vi "Teleop.vi"(10 "Match Info":T2={"Autonomous Elapsed Seconds"=0.0, "TeleOp Elapsed Seconds"=0.0, "Disabled Elapsed Seconds"=0.0, "Visited Autonomous"=FALSE, "Visited TeleOp"=FALSE, "Visited Disabled"=FALSE, "Autonomous Settings"={"Autonomous Style"=enum."Independent", "VI Refnum"=refnum}}, 11 "Call Context":T3) -> ()   [LabVIEW 2016]
doc: "This VI is called for each TeleOp packet received from the DS where the robot is not disabled. It is often used to read from the joysticks and update I/O or to update setpoints for timed control loops. It should complete and return within 20 milliseconds or it may miss DS packets."
uses:
  <vilib>/Rock Robotics/WPI/DriverStation/WPI_DriverStationDerivedRobotMode.ctl
  <vilib>/Rock Robotics/WPI/DriverStation/WPI_DriverStationMatch Info.ctl
  <vilib>/Rock Robotics/WPI/Utilities/WPI_GetSetVariantRefNum.vi
  Robot Global Data.vi
  <vilib>/Rock Robotics/WPI/Solenoid/Deprecated/WPI_SolenoidSetBool.vi
  <vilib>/addons/control/pid/pid.llb/PID (DBL).vi
  navX Library v2/navX Library v2.lvlib
  <vilib>/addons/control/pid/NI_PID_pid.lvlib
panel:
  in  "Mode":bool
  in  "output range":cluster{"output high":dbl, "output low":dbl}={"output high"=100.0, "output low"=-100.0} {"output low" format="%.2f"; "output high" format="%.2f"}
  in  "PID gains":T1={"proportional gain (Kc)"=1.0, "integral time (Ti, min)"=0.01, "derivative time (Td, min)"=0.0} {"derivative time (Td, min)" format="%.3f"; "integral time (Ti, min)" format="%.3f"; "proportional gain (Kc)" format="%.3f"}
  out "Left":dbl(graph)
  out "Right":dbl(graph)
  out "Encoder Right":dbl(graph)
  out "Encoder Left":dbl(graph)
  in  "Speed":dbl=0.5 format="%#_13g"
  out "Out Left":dbl(graph)
  out "Out Right":dbl(graph)
  out "Shooter":cluster{"Sensor Velocity":dbl, dbl, dbl}(graph)
  in  "ShooterRPM":dbl
  in  "P":dbl=0.5 format="%#_13g"
  in  "I":dbl format="%#_13g"
  in  "D":dbl format="%#_13g"
  in  "F":dbl=0.005212 format="%#_13g"
  in  "I Zone":dbl format="%#_13g"
  in  "Ramp Rate":dbl format="%#_13g"
  # "False = PID On\nTrue = PID Off\nDon't switch!!!"
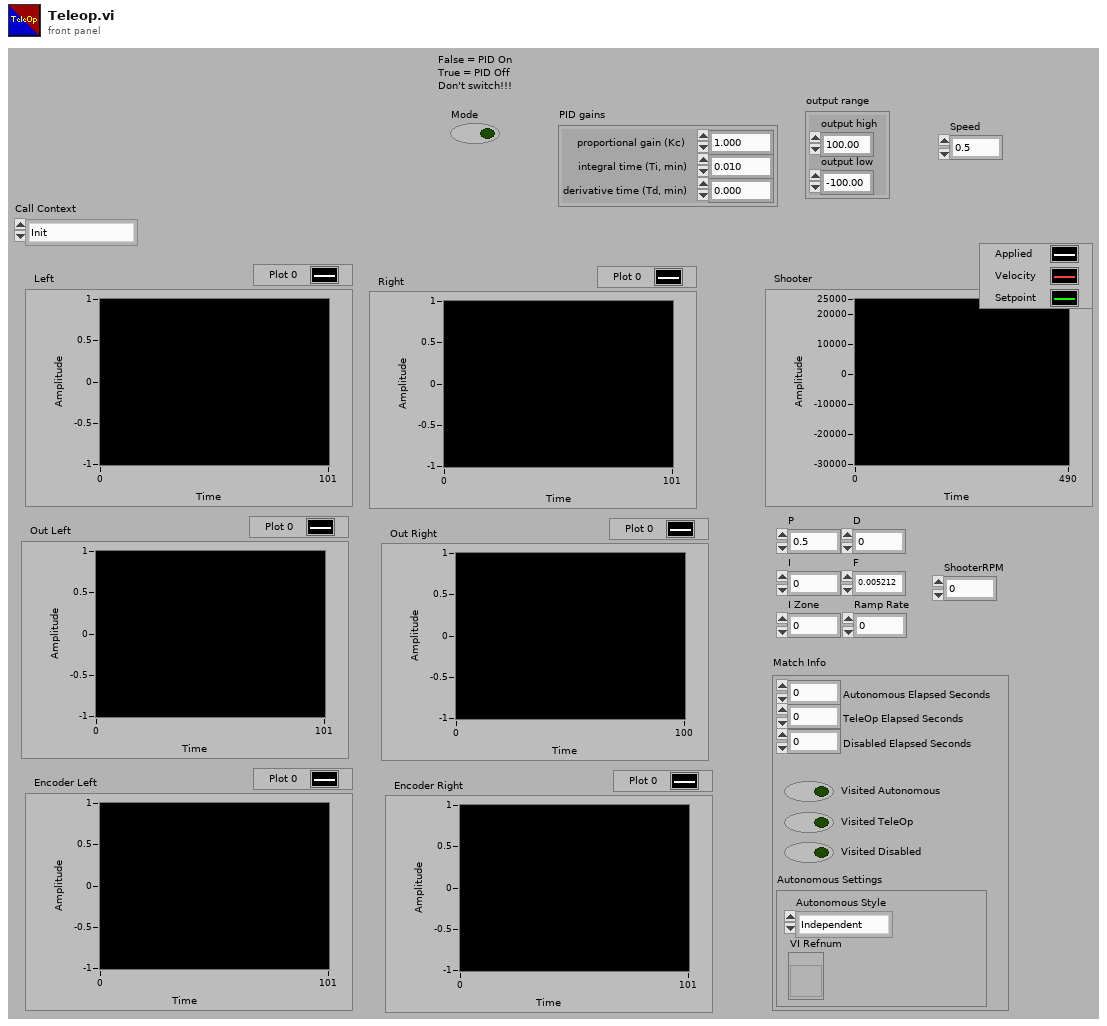
[diagram p1: front panel]
types:
  T1 = cluster{"proportional gain (Kc)":dbl, "integral time (Ti, min)":dbl, "derivative time (Td, min)":dbl}
  T2 = typedef "WPI_DriverStationMatch Info.ctl" = cluster{"Autonomous Elapsed Seconds":dbl, "TeleOp Elapsed Seconds":dbl, "Disabled Elapsed Seconds":dbl, "Visited Autonomous":bool, "Visited TeleOp":bool, "Visited Disabled":bool, "Autonomous Settings":cluster{"Autonomous Style":enum16{"Iterative", "Independent"}, "VI Refnum":refnum<vi>}}
  T3 = typedef "WPI_DriverStationDerivedRobotMode.ctl" = enum16{"Init", "Execute", "Stop"}
  T4 = typedef "WPI_SolenoidDevRef.ctl" = cluster{"DevStatus":errorcluster, "Pneumatics Control Module":u8, "Forward Solenoid Channel":T5, "Reverse Solenoid Channel":T5}
  T5 = typedef "WPI_SolenoidChannel.ctl" = enum8{"Solenoid 0", "Solenoid 1", "Solenoid 2", "Solenoid 3", "Solenoid 4", "Solenoid 5", "Solenoid 6", "Solenoid 7", "Invalid"}
  T6 = typedef "WPI_JoystickDevRef.ctl" = cluster{"Device":T7}
  T7 = typedef "WPI_JoystickDeviceEnum.ctl" = enum16{"USB 0", "USB 1", "USB 2", "USB 3", "USB 4", "USB 5"}
  T8 = cluster{"Buttons[0]":bool, "Buttons[1]":bool, "Buttons[2]":bool, "Buttons[3]":bool, "Buttons[4]":bool, "Buttons[5]":bool, "Buttons[6]":bool, "Buttons[7]":bool, "Buttons[8]":bool}
  T9 = cluster{"Axes[0]":dbl, "Axes[1]":dbl, "Axes[2]":dbl, "Axes[3]":dbl, "Axes[4]":dbl, "Axes[5]":dbl, "Axes[6]":dbl, "Axes[7]":dbl, "Axes[8]":dbl}
  T10 = typedef "navX Library v2.lvlib/Z900_navX_DeviceTypeDef.ctl" = cluster{"Interface":cluster{"Protocol":T11, "Update Rate (4Hz-100Hz)":u8, "navX Open TypeDef":variant}, "Notify Packet":refnum<notifier>, "Loop VI Refnum":refnum<vi>, "Ready to Close Occurrence Refnum":refnum<k4>}
  T11 = typedef "navX Library v2.lvlib/Z900_navX_ProtocolTypeDef.ctl" = enum16{"SERIAL", "I2C", "SPI"}
  T12 = cluster{"Velocity X":dbl, "Velocity Y":dbl, "Velocity Z":dbl, "Displacement X":dbl, "Displacement Y":dbl, "Displacement Z":dbl}
  T13 = cluster{"LinearAcceleration X":dbl, "LinearAcceleration Y":dbl, "LinearAcceleration Z":dbl}
  T14 = cluster{"Quat W":dbl, "Quat X":dbl, "Quat Y":dbl, "Quat Z":dbl}
  T15 = cluster{"Yaw":dbl, "Roll":dbl, "Pitch":dbl, "Heading":dbl, "Fused Heading":dbl}
  T16 = cluster{"Velocity X":dbl, "Velocity Y":dbl, "Velocity Z":dbl, "Displacement X":dbl, "Displacement Y":dbl, "Displacement Z":dbl, "LinearAcceleration X":dbl, "LinearAcceleration Y":dbl, "LinearAcceleration Z":dbl, "Quat W":dbl, "Quat X":dbl, "Quat Y":dbl, "Quat Z":dbl, "Yaw":dbl, "Roll":dbl, "Pitch":dbl}
  T17 = typedef "WPI_MotorControlDeviceRef.ctl" = cluster{"DeviceStatus":errorcluster, "Type":T18, "PWM":cluster{"PWM Channel":T19, "DeadBand":T20}, "CAN":cluster{"Device Number":u8, "SetOutput VI Ref":variant, "GetOutput VI Ref":variant, "Enable VI Ref":variant, "Disable VI Ref":variant, "Data":variant}, "Invert":bool}
  T18 = typedef "WPI_MotorControlType.ctl" = enum16{"PWM", "CAN"}
  T19 = typedef "FPGA_DIOPWMChannel.ctl" = enum8{"PWM 0", "PWM 1", "PWM 2", "PWM 3", "PWM 4", "PWM 5", "PWM 6", "PWM 7", "PWM 8", "PWM 9", "PWM MXP 0", "PWM MXP 1", "PWM MXP 2", "PWM MXP 3", "PWM MXP 4", "PWM MXP 5", "PWM MXP 6", "PWM MXP 7", "PWM MXP 8", "PWM MXP 9", "Invalid"}
  T20 = typedef "WPI_PWMDeadband.ctl" = cluster{"Name":string, "maxPositivePwm":i32, "minPositivePwm":i32, "centerPwm":i32, "maxNegativePwm":i32, "minNegativePwm":i32, "angularRange":u16}
  T21 = typedef "WPI_CANTalonSRX_GlobalStatus.ctl" = cluster{"Applied Throttle":dbl, "Module Enabled":bool, "CAN Error":errorcluster, "Closed Loop Error":dbl, "Forward Limit Switch Closed":bool, "Reverse Limit Switch Closed":bool, "Sensor Position":dbl, "Sensor Velocity":dbl, "Current":dbl, "Sticky Fault - Over Temp":bool, "Sticky Fault - Under Voltage":bool, "Sticky Fault - Forward Limit":bool, "Sticky Fault - Reverse Limit":bool, "Sticky Fault - Forward Soft Limit":bool, "Sticky Fault - Reverse Soft Limit":bool, "Brake is Enabled":bool, "Encoder Position":dbl, "Encoder Velocity":dbl, "Encoder Index Count":dbl, "Encoder A Pin State":bool, "Encoder B Pin State":bool, "Encoder Index Pin State":bool, "Analog In":dbl, "Analog In Velocity":dbl, "Temperature (C)":dbl, "Battery Voltage":dbl, "Control 5 Is Supported":bool, "Current Profile Slot Select":dbl, "Pos Div 8":bool, "Vel Div 4":bool, "Pulse Width Position":i32, "Pulse Width Velocity":i32, "Pulse Width Rise To Rise (us)":i32, "Pulse Width Rise To Fall (us)":i32, "Mot Prof Active Is Under Run":bool, "Mot Prof Active Has Under Run":bool, "Mot Prof Active Is Last":bool, "Mot Prof Active Velocity Only":bool, "Mot Prof Active Is Valid":bool, "Mot Prof Buffer Is Full":bool, "Mot Prof Active Profile Slot Select":i32, "Mot Prof NextID":i32, "Mot Prof Count":i32, "Mot Prof Active Velocity":dbl, "Mot Prof Active Position":dbl, "Mot Prof Output Enable":i32}
  T22 = cluster{dbl, "Sensor Velocity":dbl, "ShooterRPM":dbl}
  T23 = typedef "WPI_RobotDriveDevRef.ctl" = cluster{"DevStatus":errorcluster, "Motors[]":T17[], "Square Inputs":bool, "Max Output":dbl}
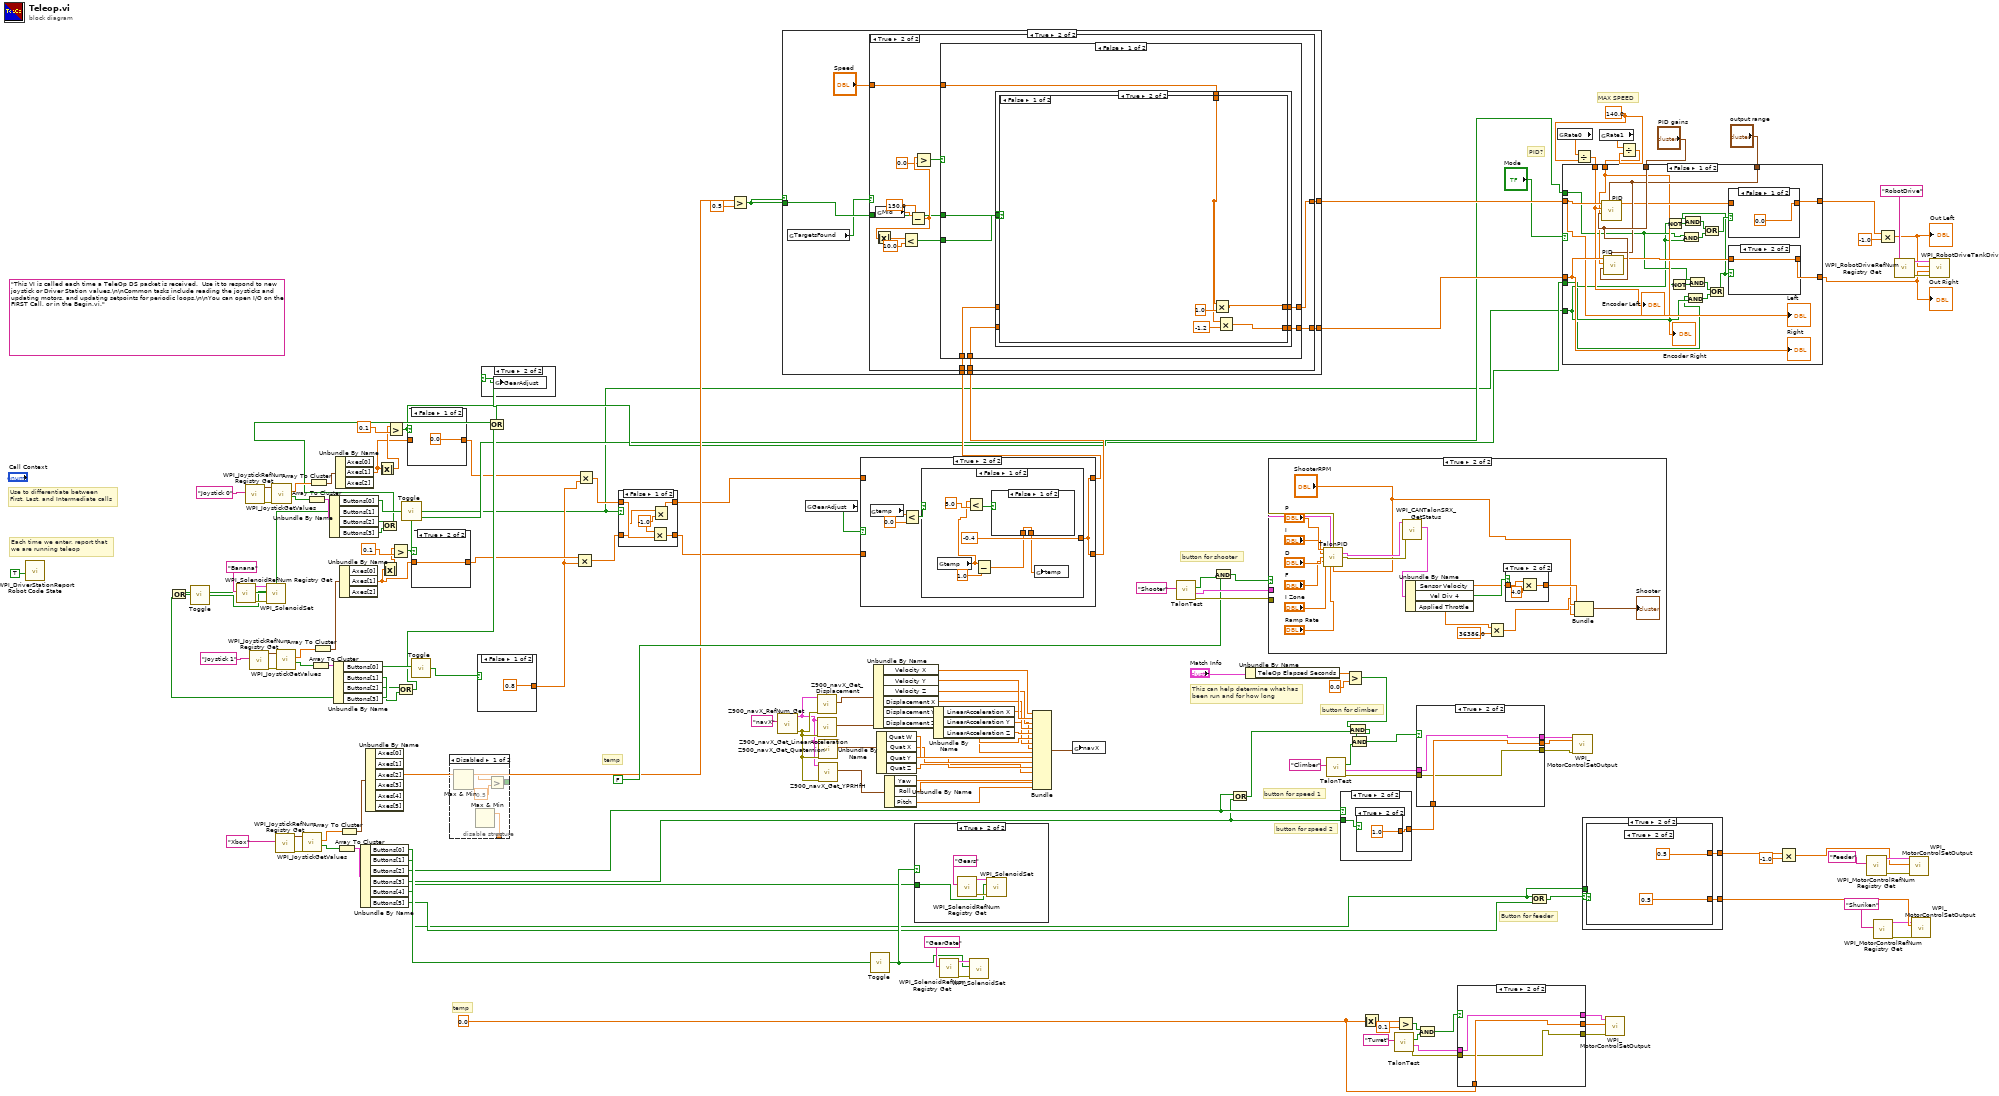
[diagram p0: block diagram]
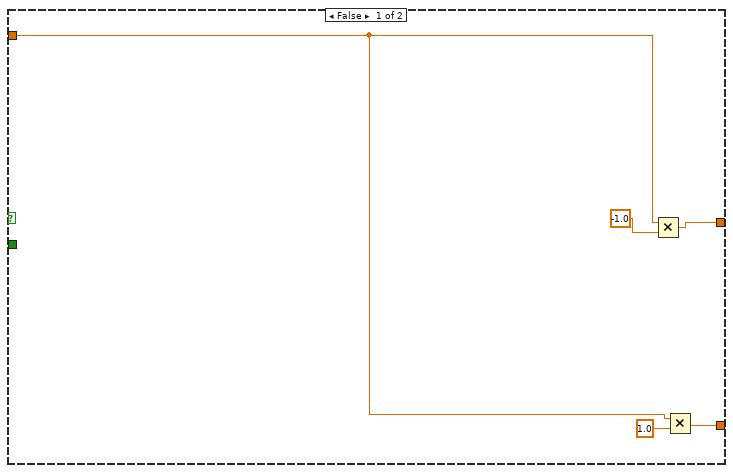
[diagram p3: hidden frame]
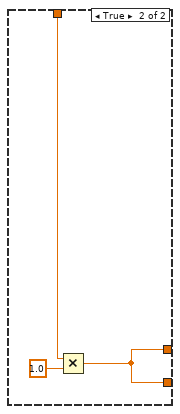
[diagram p5: hidden frame]
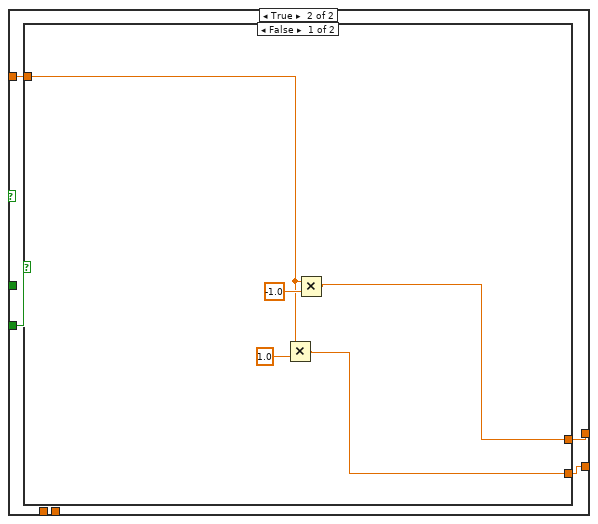
[diagram p6: hidden frame]
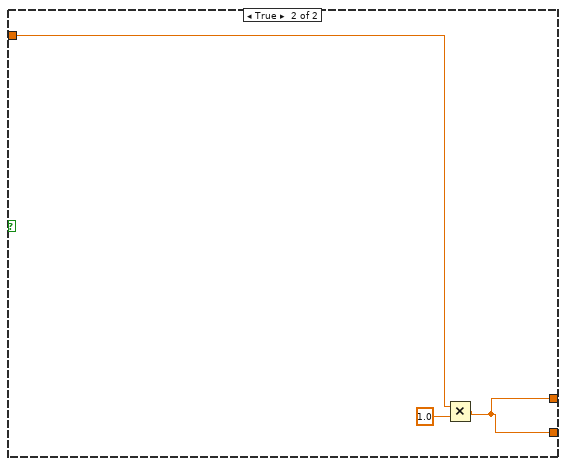
[diagram p7: hidden frame]
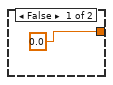
[diagram p8: hidden frame]
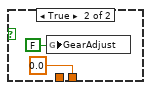
[diagram p14: hidden frame]
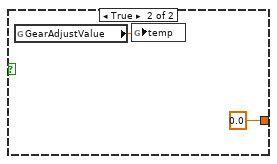
[diagram p15: hidden frame]
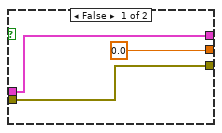
[diagram p16: hidden frame]
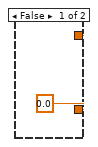
[diagram p18: hidden frame]
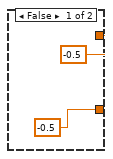
[diagram p19: hidden frame]
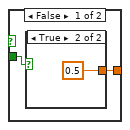
[diagram p20: hidden frame]
diagram:
  w21 = 140.0
  w34 = 0.0
  (unwired) "This VI is called each time a TeleOp DS packet is received.  Use it to respond to new joystick or Driver Station values.\n\nCommon tasks include reading the joysticks and updating motors, and updating setpoints for periodic loops.\n\nYou can open I/O on the FIRST Call, or in the Begin.vi."
  # "MAX SPEED"
  # "PID?"
  # "temp"
  # "temp"
  # "Button for feeder"
  # "button for speed 2"
  # "button for speed 1"
  # "button for climber"
  # "button for shooter"
  # "Each time we enter, report that\nwe are running teleop"
  # "Use to differentiate between\nFirst, Last, and Intermediate calls"
  # "This can help determine what has\nbeen run and for how long"
  n1 = call <vilib>:"WPI_DriverStationReport Robot Code State.vi"("TeleOp"=TRUE ("Autonomous")) -> ()  [unwired: 10 in, 1 out]
  n2 = call <vilib>:"WPI_SolenoidRefNum Registry Get.vi"("refnum name"="Banana") -> ("error out"=w59:errorcluster, "SolenoidDevRef"=w58:T4)  [unwired: 9 in]
  n3 = call <vilib>:"WPI_JoystickRefNum Registry Get.vi"("refnum name"="Joystick 0") -> ("error out"=w155:errorcluster, "JoystickDevRef"=w154:T6)  [unwired: 9 in]
  n4 = call <vilib>:"WPI_JoystickRefNum Registry Get.vi"("refnum name"="Joystick 1") -> ("error out"=w147:errorcluster, "JoystickDevRef"=w146:T6)  [unwired: 9 in]
  n5 = call <vilib>:"WPI_JoystickGetValues.vi"("error in (no error)"=w155, "JoystickDevRef"=w154) -> ("Buttons"=w151:bool[], "Axes"=w152:dbl[])  [unwired: 5 in, 3 out]
  n6 = call <vilib>:"WPI_JoystickRefNum Registry Get.vi"("refnum name"="Xbox") -> ("error out"=w88:errorcluster, "JoystickDevRef"=w87:T6)  [unwired: 9 in]
  n7 = call <vilib>:"WPI_JoystickGetValues.vi"("error in (no error)"=w147, "JoystickDevRef"=w146) -> ("Buttons"=w143:bool[], "Axes"=w144:dbl[])  [unwired: 5 in, 3 out]
  n8 = call <vilib>:"WPI_JoystickGetValues.vi"("error in (no error)"=w88, "JoystickDevRef"=w87) -> ("Buttons"=w84:bool[], "Axes"=w85:dbl[])  [unwired: 5 in, 3 out]
  n9 = Array To Cluster(array=w151) -> (cluster=w149:T8)
  n10 = Array To Cluster(array=w152) -> (cluster=w150:T9)
  n11 = Array To Cluster(array=w143) -> (cluster=w141:T8)
  n12 = Array To Cluster(array=w144) -> (cluster=w142:T9)
  n13 = Unbundle By Name(w149) -> ("Buttons[0]"=w135:bool, "Buttons[1]"=w55:bool, "Buttons[2]"=w40:bool, "Buttons[3]"=w39:bool)
  n14 = Unbundle By Name(w141) -> ("Buttons[0]"=w134:bool, "Buttons[1]"=w54:bool, "Buttons[2]"=w42:bool, "Buttons[3]"=w41:bool)
  n15 = Or(x=w55, y=w54) -> (x .or. y?=w56:bool)
  n16 = call "Toggle.vi"("Input"=w56) -> ("Output"=w53:bool)
  n17 = call-poly <vilib>:"WPI_SolenoidSet.vi"("error in (no error)"=w59, "Value"=w53, "SolenoidDevRef"=w58) -> ()  [unwired: 7 in, 2 out]
  n18 = Unbundle By Name(w150) -> ("Axes[1]"=w136:dbl)  [unwired: 2 out]
  n19 = Array To Cluster(array=w84) -> (cluster=w82:T8)
  n20 = Unbundle By Name(w142) -> ("Axes[1]"=w138:dbl)  [unwired: 2 out]
  n21 = Array To Cluster(array=w85) -> (cluster=w83:T9)
  n22 = Unbundle By Name(w82) -> ("Buttons[0]"=w81:bool, "Buttons[1]"=w80:bool, "Buttons[2]"=w79:bool, "Buttons[3]"=w78:bool, "Buttons[4]"=w75:bool, "Buttons[5]"=w76:bool)
  n23 = Unbundle By Name(w83) -> ("Axes[2]"=w32:dbl)  [unwired: 5 out]
  n24 = Absolute Value(x=w136) -> (abs(x)=w137:dbl)
  n25 = Or(x=w40, y=w39) -> (x .or. y?=w38:bool)
  n26 = Absolute Value(x=w138) -> (abs(x)=w139:dbl)
  n27 = Greater?(x=w137, y=0.1 ("x")) -> (0:w11:bool)
  n28 = Greater?(x=w139, y=0.1 ("x")) -> (0:w10:bool)
  n29 = Or(x=w42, y=w41) -> (x .or. y?=w37:bool)
  n30 = call "Toggle.vi"("Input"=w135) -> ("Output"=w1:bool)
  n31 = case shown="False" w11 {
    tunnel: w136 -> [_ w158]
    tunnel: [0.0 w158] -> w6
    frame False {
    }
    frame True {
    }
  }
  n32 = case shown="True" w10 {
    tunnel: w138 -> [_ w160]
    tunnel: [0.0 w160] -> w8
    frame False {
    }
    frame True {
    }
  }
  n33 = call "Toggle.vi"("Input"=w134) -> ("Output"=w133:bool)
  n34 = disable-structure shown="Disabled" {
    disable-tunnel: [w162 _] -> _
    disable-tunnel: [w161 _] -> _
    frame Disabled {
      n35 = Max & Min() -> (max(x,y)=w164:dbl)  [unwired: 2 in, 1 out]
      n36 = Max & Min() -> (max(x,y)=w161:dbl)  [unwired: 2 in, 1 out]
      n37 = Greater?(x=w164, y=0.5) -> (0:w162:bool)
    }
    frame Enabled {
    }
  }
  n38 = case shown="False" w133 {
    tunnel: [0.8 1.0] -> w7
    frame False {
    }
    frame True {
    }
  }
  n39 = Or(x=w38, y=w37) -> (x .or. y?=w35:bool)
  n40 = case shown="True" w35 {
    selector: w35 -> [_ w167]
    frame False {
    }
    frame True {
      n41 = global write "Robot Global Data.vi" "GearAdjust"(w167) -> ()
    }
  }
  n42 = Multiply(x=w8, y=w7) -> (x*y=w4:dbl)
  n43 = Multiply(x=w6, y=w7) -> (x*y=w5:dbl)
  n44 = case shown="False" w1 {
    tunnel: w5 -> [w169 w174]
    tunnel: w4 -> [w168 w173]
    tunnel: [w172 w174] -> w3
    tunnel: [w171 w173] -> w2
    frame False {
      w170 = -1.0
      n45 = Multiply(x=w170, y=w169) -> (x*y=w171:dbl)
      n46 = Multiply(x=w168, y=w170) -> (x*y=w172:dbl)
    }
    frame True {
    }
  }
  n47 = Greater?(x=w32, y=0.5) -> (0:w9:bool)
  n48 = call "Z900_navX_RefNum_Get.vi"("refnum name"="navX") -> ("error out"=w131:errorcluster, "navX Device"=w130:T10)  [unwired: 9 in]
  n49 = global read "Robot Global Data.vi" "GearAdjust"() -> (w36:bool)
  n50 = call "Z900_navX_Get_Displacement.vi"("error in (no error)"=w131, "navX Device"=w130) -> ("Displacement"=w126:T12)  [unwired: 6 in, 3 out]
  n51 = call "Z900_navX_Get_LinearAcceleration.vi"("error in (no error)"=w131, "navX Device"=w130) -> ("Linear Acceleration"=w127:T13)  [unwired: 6 in, 3 out]
  n52 = call "Z900_navX_Get_Quaternion.vi"("error in (no error)"=w131, "navX Device"=w130) -> ("Quaternion"=w128:T14)  [unwired: 6 in, 3 out]
  n53 = call "Z900_navX_Get_YPRHfH.vi"("error in (no error)"=w131, "navX Device"=w130) -> ("YRPHfH"=w129:T15)  [unwired: 6 in, 3 out]
  n54 = case shown="True" w36 {
    tunnel: w3 -> [w176 _]
    tunnel: w2 -> [w175 _]
    tunnel: [w176 w177] -> w27
    tunnel: [w175 w177] -> w26
    frame False {
    }
    frame True {
      n55 = global read "Robot Global Data.vi" "temp"() -> (w180:dbl)
      n56 = Less?(x=w180, y=0.0) -> (x < y?=w178:bool)
      n57 = case shown="False" w178 {
        tunnel: [-0.4 0.0] -> w177
        frame False {
          n58 = global read "Robot Global Data.vi" "temp"() -> (w183:dbl)
          n59 = Less?(x=w183, y=5.0 ("x")) -> (x < y?=w184:bool)
          n60 = Subtract(x=w183, y=1.0) -> (x-y=w181:dbl)
          n61 = case shown="False" w184 {
            tunnel: [w188 0.0] -> w182
            tunnel: w181 -> [w188 _]
            frame False {
            }
            frame True {
              n62 = global write "Robot Global Data.vi" "GearAdjust"(FALSE) -> ()
            }
          }
          n63 = global write "Robot Global Data.vi" "temp"(w182) -> ()
        }
        frame True {
          n64 = global read "Robot Global Data.vi" "GearAdjustValue"() -> (w192:dbl)
          n65 = global write "Robot Global Data.vi" "temp"(w192) -> ()
        }
      }
    }
  }
  n66 = case shown="True" w9 {
    tunnel: w27 -> [w194 w201]
    tunnel: w26 -> [w193 w200]
    tunnel: w9 -> [_ w198]
    tunnel: [w194 w197] -> w17
    tunnel: [w193 w196] -> w16
    frame False {
    }
    frame True {
      n67 = global read "Robot Global Data.vi" "TargetsFound"() -> (w195:bool)
      n68 = case shown="True" w195 {
        tunnel: w201 -> [_ w215]
        tunnel: w200 -> [_ w214]
        tunnel: [w204 w213] -> w196
        tunnel: [w205 w212] -> w197
        tunnel: w198 -> [_ w208]
        tunnel: "Speed" -> [w202 w207]
        frame False {
          n69 = Multiply(x=w202, y=-1.0) -> (x*y=w205:dbl)
          n70 = Multiply(x=w202, y=1.0) -> (x*y=w204:dbl)
        }
        frame True {
          n71 = global read "Robot Global Data.vi" "Mid"() -> (w220:dbl)
          n72 = Subtract(x=w220, y=150.0) -> (x-y=w210:dbl)
          n73 = Absolute Value(x=w210) -> (abs(x)=w218:dbl)
          n74 = Less?(x=w218, y=10.0) -> (x < y?=w216:bool)
          n75 = Greater?(x=w210, y=0.0) -> (0:w211:bool)
          n76 = case shown="False" w211 {
            tunnel: w216 -> [w227 w245]
            tunnel: w215 -> [w226 _]
            tunnel: w214 -> [w225 _]
            tunnel: [w224 w243] -> w213
            tunnel: [w223 w244] -> w212
            tunnel: w208 -> [w222 _]
            tunnel: w207 -> [w221 w242]
            frame False {
              n77 = case shown="True" w222 {
                tunnel: w227 -> [_ w233]
                tunnel: w226 -> [w229 _]
                tunnel: w225 -> [w228 _]
                tunnel: [w229 w232] -> w223
                tunnel: [w228 w231] -> w224
                tunnel: w221 -> [_ w230]
                frame False {
                }
                frame True {
                  n78 = case shown="False" w233 {
                    tunnel: [w238 w241] -> w232
                    tunnel: [w236 w241] -> w231
                    tunnel: w230 -> [w234 w239]
                    frame False {
                      n79 = Multiply(x=w234, y=1.0) -> (x*y=w238:dbl)
                      n80 = Multiply(x=w234, y=-1.2) -> (x*y=w236:dbl)
                    }
                    frame True {
                      n81 = Multiply(x=w239, y=1.0) -> (x*y=w241:dbl)
                    }
                  }
                }
              }
            }
            frame True {
              n82 = case shown="False" w245 {
                tunnel: [w250 w253] -> w244
                tunnel: [w248 w253] -> w243
                tunnel: w242 -> [w246 w251]
                frame False {
                  n83 = Multiply(x=w246, y=1.0) -> (x*y=w248:dbl)
                  n84 = Multiply(x=w246, y=-1.0) -> (x*y=w250:dbl)
                }
                frame True {
                  n85 = Multiply(x=w251, y=1.0) -> (x*y=w253:dbl)
                }
              }
            }
          }
        }
      }
    }
  }
  n86 = call "Toggle.vi"("Input"=w81) -> ("Output"=w89:bool)
  n87 = Unbundle By Name(w126) -> ("Velocity X"=w125:dbl, "Velocity Y"=w124:dbl, "Velocity Z"=w123:dbl, "Displacement X"=w122:dbl, "Displacement Y"=w121:dbl, "Displacement Z"=w120:dbl)
  n88 = Unbundle By Name(w128) -> ("Quat W"=w116:dbl, "Quat X"=w115:dbl, "Quat Y"=w114:dbl, "Quat Z"=w113:dbl)
  n89 = Unbundle By Name(w129) -> ("Yaw"=w112:dbl, "Roll"=w111:dbl, "Pitch"=w110:dbl)
  n90 = case shown="True" w89 {
    tunnel: w80 -> [_ w254]
    frame False {
    }
    frame True {
      n91 = call <vilib>:"WPI_SolenoidRefNum Registry Get.vi"("refnum name"="Gears") -> ("error out"=w257:errorcluster, "SolenoidDevRef"=w256:T4)  [unwired: 9 in]
      n92 = call-poly <vilib>:"WPI_SolenoidSet.vi"("error in (no error)"=w257, "Value"=w254, "SolenoidDevRef"=w256) -> ()  [unwired: 7 in, 2 out]
    }
  }
  n93 = Unbundle By Name(w127) -> ("LinearAcceleration X"=w119:dbl, "LinearAcceleration Y"=w118:dbl, "LinearAcceleration Z"=w117:dbl)
  n94 = call <vilib>:"WPI_SolenoidRefNum Registry Get.vi"("refnum name"="GearGate") -> ("error out"=w92:errorcluster, "SolenoidDevRef"=w91:T4)  [unwired: 9 in]
  n95 = call-poly <vilib>:"WPI_SolenoidSet.vi"("error in (no error)"=w92, "Value"=w89, "SolenoidDevRef"=w91) -> ()  [unwired: 7 in, 2 out]
  n96 = Bundle("Velocity X"=w125, "Velocity Y"=w124, "Velocity Z"=w123, "Displacement X"=w122, "Displacement Y"=w121, "Displacement Z"=w120, "LinearAcceleration X"=w119, "LinearAcceleration Y"=w118, "LinearAcceleration Z"=w117, "Quat W"=w116, "Quat X"=w115, "Quat Y"=w114, "Quat Z"=w113, "Yaw"=w112, "Roll"=w111, "Pitch"=w110) -> (w109:T16)  [unwired: 1 in]
  n97 = global write "Robot Global Data.vi" "navX"(w109) -> ()
  n98 = call "TalonTest.vi"("Name"="Shooter") -> ("Output"=w103:bool, "Ref"=w107:T17, "error out"=w106:errorcluster)  [unwired: 7 in]
  n99 = And(x=FALSE, y=w103) -> (x .and. y?=w104:bool)
  n100 = Or(x=w79, y=w78) -> (x .or. y?=w77:bool)
  n101 = Unbundle By Name("Match Info") -> ("TeleOp Elapsed Seconds"=w99:dbl)
  n102 = case shown="True" w104 {
    tunnel: w107 -> [_ w262]
    tunnel: w106 -> [_ w261]
    frame False {
    }
    frame True {
      n103 = call "TalonPID.vi"("P"="P", "Ref In"=w262, "Error in"=w261, "I"="I", "D"="D", "F"="F", "I Zone"="I Zone", "Ramp Rate"="Ramp Rate", "Output"="ShooterRPM") -> ("Ref Out"=w260:T17, "error out"=w259:errorcluster)  [unwired: 5 in]
      n104 = call <vilib>:"WPI_CANTalonSRX_GetStatus.vi"("error in (no error)"=w259, "CAN Talon SRX Ref"=w260) -> ("Talon SRX Status"=w276:T21)  [unwired: 7 in, 2 out]
      n105 = Unbundle By Name(w276) -> ("Sensor Velocity"=w274:dbl, "Vel Div 4"=w275:bool, "Applied Throttle"=w271:dbl)
      n106 = Multiply(x=w271, y=36386.0) -> (x*y=w270:dbl)
      n107 = case shown="True" w275 {
        tunnel: w274 -> [w277 w279]
        tunnel: [w277 w280] -> w269
        frame False {
        }
        frame True {
          n108 = Multiply(x=w279, y=4.0) -> (x*y=w280:dbl)
        }
      }
      n109 = Bundle(w270, "Sensor Velocity"=w269, "ShooterRPM"="ShooterRPM") -> (→"Shooter":T22)  [unwired: 1 in]
    }
  }
  n110 = call "TalonTest.vi"("Name"="Climber") -> ("Output"=w101:bool, "Ref"=w95:T17, "error out"=w94:errorcluster)  [unwired: 7 in]
  n111 = case shown="True" w79 {
    tunnel: [w282 w286] -> w93
    tunnel: w78 -> [w281 w285]
    frame False {
      n112 = case shown="True" w281 {
        tunnel: [0.0 0.5] -> w282
        frame False {
        }
        frame True {
        }
      }
    }
    frame True {
      n113 = case shown="True" w285 {
        tunnel: [0.75 1.0] -> w286
        frame False {
        }
        frame True {
        }
      }
    }
  }
  n114 = Greater?(x=w99, y=0.0) -> (0:w97:bool)
  n115 = And(x=w97, y=w77) -> (x .and. y?=w102:bool)
  n116 = And(x=w102, y=w101) -> (x .and. y?=w96:bool)
  n117 = Absolute Value(x=w34) -> (abs(x)=w68:dbl)
  n118 = call "TalonTest.vi"("Name"="Turret") -> ("Output"=w72:bool, "Ref"=w70:T17, "error out"=w69:errorcluster)  [unwired: 7 in]
  n119 = Greater?(x=w68, y=0.1) -> (0:w66:bool)
  n120 = case shown="True" w96 {
    tunnel: w95 -> [w290 w294]
    tunnel: w94 -> [w289 w292]
    tunnel: w93 -> [_ w293]
    tunnel: [w290 w294] -> w61
    tunnel: [0.0 w293] -> w62
    tunnel: [w289 w292] -> w60
    frame False {
    }
    frame True {
    }
  }
  n121 = And(x=w66, y=w72) -> (x .and. y?=w71:bool)
  n122 = case shown="True" w71 {
    tunnel: w70 -> [w296 w300]
    tunnel: w69 -> [w295 w298]
    tunnel: w34 -> [_ w299]
    tunnel: [w296 w300] -> w65
    tunnel: [0.0 w299] -> w64
    tunnel: [w295 w298] -> w63
    frame False {
    }
    frame True {
    }
  }
  n123 = Or(x=w75, y=w76) -> (x .or. y?=w74:bool)
  n124 = global read "Robot Global Data.vi" "Rate0"() -> (w23:dbl)
  n125 = call <vilib>:"WPI_MotorControlSetOutput.vi"("error in (no error)"=w60, "Output"=w62, "MotorControlDevRef"=w61) -> ()  [unwired: 6 in, 3 out]
  n126 = Divide(x=w23, y=w21) -> (x/y=w20:dbl)
  n127 = case shown="True" w74 {
    tunnel: w75 -> [_ w304]
    tunnel: [w301 w303] -> w45
    tunnel: [w301 w302] -> w52
    frame False {
      w301 = 0.0
    }
    frame True {
      n128 = case shown="True" w304 {
        tunnel: [-0.5 ("Output") 0.5 ("Output")] -> w303
        tunnel: [-0.5 ("Output") 0.5 ("Output")] -> w302
        frame False {
        }
        frame True {
        }
      }
    }
  }
  n129 = global read "Robot Global Data.vi" "Rate1"() -> (w22:dbl)
  n130 = call <vilib>:"WPI_MotorControlSetOutput.vi"("error in (no error)"=w63, "Output"=w64, "MotorControlDevRef"=w65) -> ()  [unwired: 6 in, 3 out]
  n131 = Divide(x=w22, y=w21) -> (x/y=w19:dbl)
  n132 = case shown="False" "Mode" {
    tunnel: w17 -> [w322 w334]
    tunnel: w16 -> [w323 w335]
    tunnel: w20 -> [w321 _]
    tunnel: w19 -> [w320 _]
    tunnel: "PID gains" -> [w329 _]
    tunnel: "output range" -> [w328 _]
    tunnel: w11 -> [w312 _]
    tunnel: w10 -> [w310 _]
    tunnel: [w324 w335] -> w14
    tunnel: [w325 w334] -> w15
    tunnel: w1 -> [w311 _]
    frame False {
      n133 = call-poly <vilib>:"PID.vi"("output range"=w328, "PID gains"=w329, "process variable"=w321, "setpoint"=w322) -> ("output"=w326:dbl)  [unwired: 6 in, 1 out]
      n134 = call-poly <vilib>:"PID.vi"("output range"=w328, "PID gains"=w329, "process variable"=w320, "setpoint"=w323) -> ("output"=w327:dbl)  [unwired: 6 in, 1 out]
      n135 = Not(x=w311) -> (.not. x?=w317:bool)
      n136 = Not(x=w311) -> (.not. x?=w314:bool)
      n137 = And(x=w312, y=w311) -> (x .and. y?=w319:bool)
      n138 = And(x=w310, y=w311) -> (x .and. y?=w313:bool)
      n139 = And(x=w312, y=w314) -> (x .and. y?=w315:bool)
      n140 = Or(x=w315, y=w313) -> (x .or. y?=w309:bool)
      n141 = And(x=w309, y=w317) -> (x .and. y?=w318:bool)
      n142 = Or(x=w318, y=w319) -> (x .or. y?=w316:bool)
      n143 = case shown="False" w316 {
        tunnel: w326 -> [_ w333]
        tunnel: [0.0 w333] -> w325
        frame False {
        }
        frame True {
        }
      }
      n144 = case shown="True" w309 {
        tunnel: w327 -> [_ w331]
        tunnel: [0.0 w331] -> w324
        frame False {
        }
        frame True {
        }
      }
      "Left" <- w322
      "Right" <- w323
      "Encoder Right" <- w320
      "Encoder Left" <- w321
    }
    frame True {
    }
  }
  "Out Right" <- w14
  n145 = Multiply(x=w45, y=-1.0) -> (x*y=w43:dbl)
  n146 = call <vilib>:"WPI_MotorControlRefNum Registry Get.vi"("refnum name"="Feeder") -> ("error out"=w46:errorcluster, "MotorControlDevRef"=w47:T17)  [unwired: 9 in]
  n147 = call <vilib>:"WPI_MotorControlRefNum Registry Get.vi"("refnum name"="Shuriken") -> ("error out"=w48:errorcluster, "MotorControlDevRef"=w49:T17)  [unwired: 9 in]
  n148 = Multiply(x=w15, y=-1.0) -> (x*y=w25:dbl)
  "Out Left" <- w25
  n149 = call <vilib>:"WPI_RobotDriveRefNum Registry Get.vi"("refnum name"="RobotDrive") -> ("error out"=w31:errorcluster, "RobotDriveDevRef"=w30:T23)  [unwired: 9 in]
  n150 = call <vilib>:"WPI_MotorControlSetOutput.vi"("error in (no error)"=w46, "Output"=w43, "MotorControlDevRef"=w47) -> ()  [unwired: 6 in, 3 out]
  n151 = call <vilib>:"WPI_MotorControlSetOutput.vi"("error in (no error)"=w48, "Output"=w52, "MotorControlDevRef"=w49) -> ()  [unwired: 6 in, 3 out]
  n152 = call <vilib>:"WPI_RobotDriveTankDrive.vi"("error in (no error)"=w31, "Right axis value"=w14, "Left axis value"=w25, "RobotDriveDevRef"=w30) -> ()  [unwired: 5 in, 3 out]
